vi "_ConnectorPaneEditor_SetNewControlName.vi"(8 "error in (no error)":errorcluster, 9 "Row":i32, 10 "NewString":string, 11 "ConnectorPaneEditor in":refnum<class "_ConnectorPaneEditor.lvclass">) -> (0 "error out":errorcluster, 3 "ConnectorPaneEditor out":refnum<class "_ConnectorPaneEditor.lvclass">)   [LabVIEW 2014, in "_ConnectorPaneEditor.lvclass"]
uses:
  _ConnectorPaneEditor.lvclass
  _ConnectorPaneEditor.lvclass/_ConnectorPaneEditor.ctl
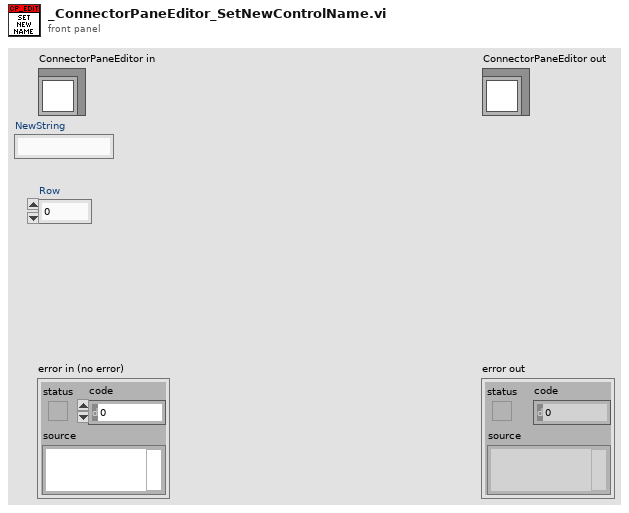
[diagram p1: front panel]
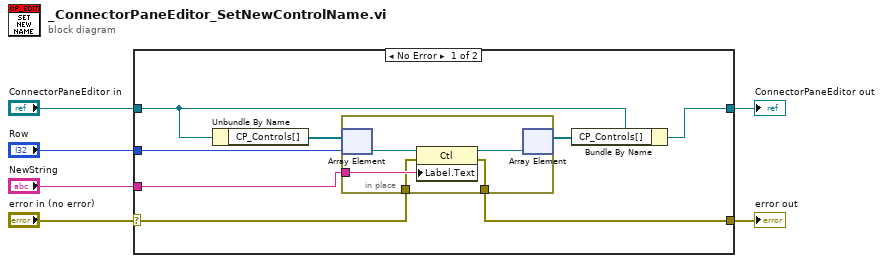
[diagram p0: block diagram]
diagram:
  n1 = case shown="No Error" "error in (no error)" {
    selector: "error in (no error)" -> [w11 w21]
    tunnel: [w10 w21] -> w5
    tunnel: [w7 w20] -> w3
    tunnel: "ConnectorPaneEditor in" -> [w8 w20]
    tunnel: "NewString" -> [w12 _]
    tunnel: "Row" -> [w13 _]
    frame No Error {
      n2 = Unbundle By Name(w8) -> ("CP_Controls[]"=w14:refnum<vi>[])
      n3 = in-place {
        in-place-border: w12 -> [w18]
        in-place-border: w11 -> [w17]
        in-place-border: [w16] -> w10
        n4 = in-place-array #1(w14, w13) -> (w19:refnum<vi>)
        n5 = property class="Ctl"(reference=w19, error in=w17, "Label.Text"=w18) -> (reference out=w15:refnum<vi>, error out=w16:errorcluster)
        n6 = in-place-array #1(w15) -> (w9:refnum<vi>[])  [unwired: 1 out]
      }
      n7 = Bundle By Name(cluster=w8, "CP_Controls[]"=w9) -> (w7:refnum<class "_ConnectorPaneEditor.lvclass">)
    }
    frame Error {
    }
  }
  "error out" <- w5
  "ConnectorPaneEditor out" <- w3
